vi "Calculate N Cubes.vi"(8 "error in (no error)":errorcluster, 11 "Cube in":refnum<class "Cube.lvclass">) -> (0 "error out":errorcluster, 2 "N Cubes":i64, 3 "Cube out":refnum<class "Cube.lvclass">)   [LabVIEW 2019, in "22.lvlib" / "Cube.lvclass"]
uses:
  Cube.lvclass
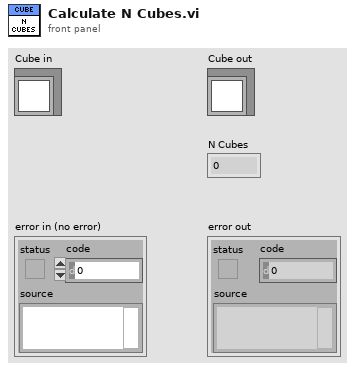
[diagram p1: front panel]
types:
  T1 = cluster{"xmin":i64, "xmax":i64, "ymin":i64, "ymax":i64, "zmin":i64, "zmax":i64}
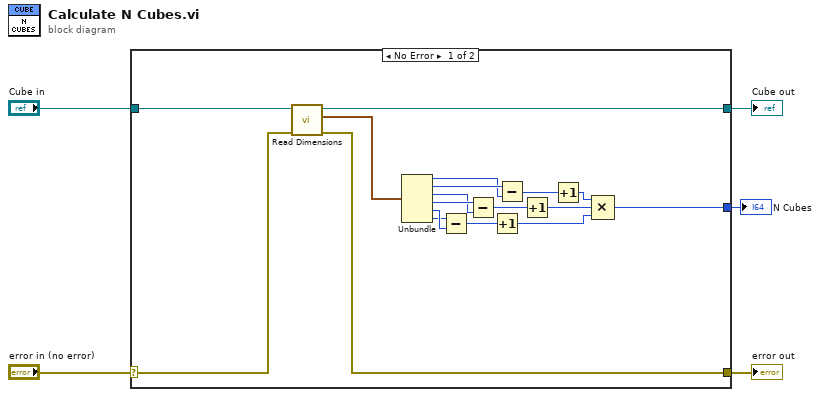
[diagram p0: block diagram]
diagram:
  n1 = case shown="No Error" "error in (no error)" {
    selector: "error in (no error)" -> [w21 w25]
    tunnel: [w20 w25] -> w4
    tunnel: [w23 w24] -> w2
    tunnel: "Cube in" -> [w22 w24]
    tunnel: [w6 _] -> w1
    frame No Error {
      n2 = call-dynamic "Read Dimensions.vi"("error in (no error)"=w21, "Cube in"=w22) -> ("error out"=w20:errorcluster, "Dimensions"=w19:T1, "Cube out"=w23:refnum<class "Cube.lvclass">)  [unwired: 7 in]
      n3 = Unbundle(w19) -> ("xmin"=w17:i64, "xmax"=w18:i64, "ymin"=w15:i64, "ymax"=w16:i64, "zmin"=w14:i64, "zmax"=w13:i64)
      n4 = Subtract(x=w13, y=w14) -> (x-y=w10:i64)
      n5 = Subtract(x=w16, y=w15) -> (x-y=w11:i64)
      n6 = Increment(x=w10) -> (x+1=w7:i64)
      n7 = Subtract(x=w18, y=w17) -> (x-y=w12:i64)
      n8 = Increment(x=w11) -> (x+1=w8:i64)
      n9 = Increment(x=w12) -> (x+1=w9:i64)
      n10 = Compound Arithmetic op=MULTIPLY(w9, w8, w7) -> (w6:i64)
    }
    frame Error {
    }
  }
  "error out" <- w4
  "Cube out" <- w2
  "N Cubes" <- w1
